vi "test_Error Code and Message Status Channels by Generating TCP Errors.vi"(8 "error in (no error)":errorcluster, 11 "TestCase in":refnum<class "Instrument Addon Error System Tests.lvclass">) -> (0 "error out":errorcluster, 3 "TestCase out":refnum<class "Instrument Addon Error System Tests.lvclass">)   [LabVIEW 2019, in "Instrument Addon Error System Tests.lvclass"]
uses:
  Instrument Addon Error System Tests.lvclass
  C:/Program Files (x86)/National Instruments/LabVIEW 2019/vi.lib/NI/VeriStand Custom Device Testing Tools/VeriStandTestCase/VeriStandTestCase.lvclass
  <vilib>/NI VeriStand/Execution/Workspace/NI VeriStand - Set Multiple Channel Values.vi
  <vilib>/NI VeriStand/Execution/Workspace/NI VeriStand - Get Single Channel Value.vi
  <vilib>/addons/_JKI Toolkits/VI Tester/TestCase.llb/TestCase.lvclass
  <vilib>/NI VeriStand/Execution/Workspace/NI_VS Workspace ExecutionAPI.lvlib
  C:/Program Files (x86)/National Instruments/LabVIEW 2019/vi.lib/addons/_JKI Toolkits/VI Tester/TestCase.llb/TestCase.lvclass
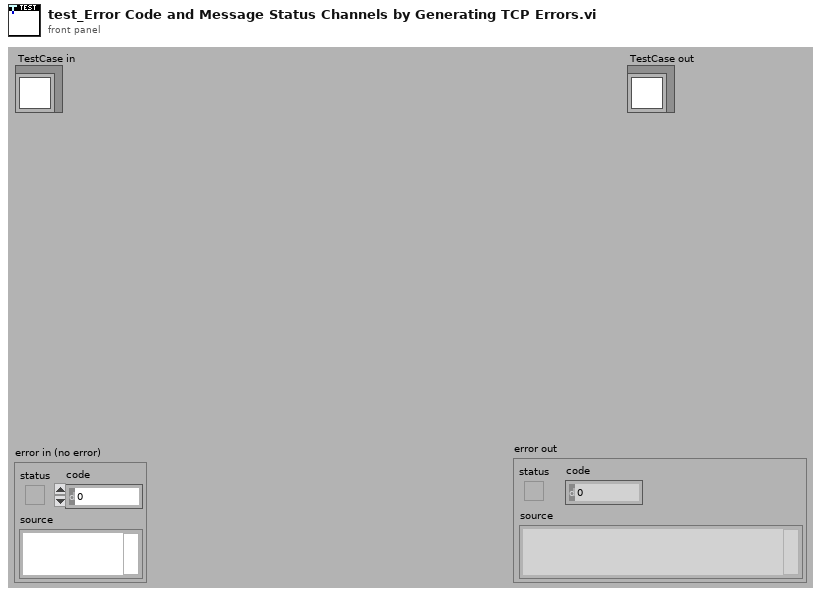
[diagram p1: front panel]
types:
  T1 = typedef "NI_VS Workspace ExecutionAPI.lvlib/WorkspaceAPI.ctl" = refnum<k24>
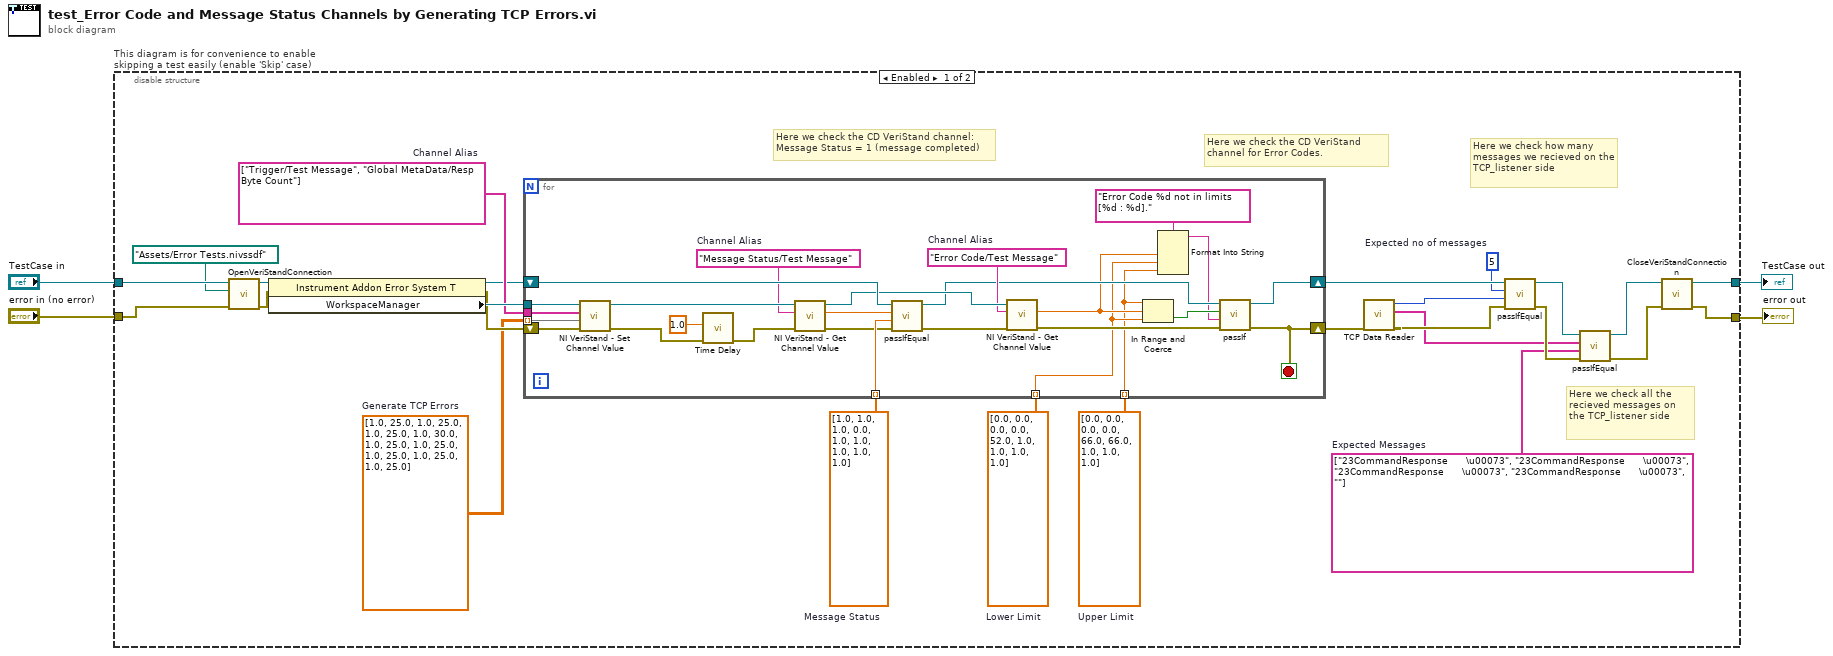
[diagram p0: block diagram]
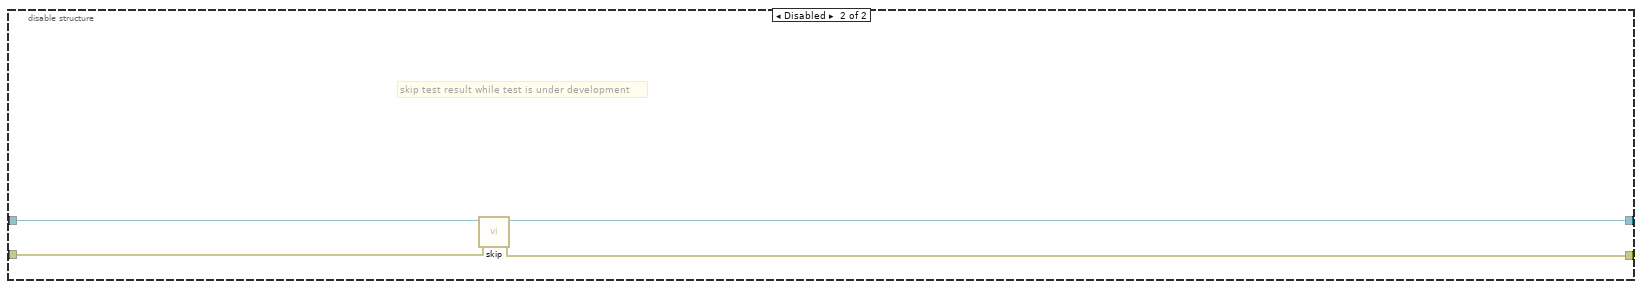
[diagram p2: hidden frame]
diagram:
  n1 = disable-structure "This diagram is for convenience to enable skipping a test easily (enable 'Skip' case)" shown="Enabled" {
    disable-tunnel: "TestCase in" -> [w28 w60]
    disable-tunnel: [w29 w58] -> w1
    disable-tunnel: [w30 w59] -> w3
    disable-tunnel: "error in (no error)" -> [w26 w57]
    frame Enabled {
      w5 = dbl[] [0.0, 0.0, 0.0, 0.0, 52.0, 1.0, 1.0, 1.0, 1.0]  # Lower Limit
      w6 = dbl[] [0.0, 0.0, 0.0, 0.0, 66.0, 66.0, 1.0, 1.0, 1.0]  # Upper Limit
      w7 = dbl[] [1.0, 1.0, 1.0, 0.0, 1.0, 1.0, 1.0, 1.0, 1.0]  # Message Status
      w8 = dbl[][] [[1.0, 25.0], [1.0, 25.0], [1.0, 25.0], [1.0, 30.0], [1.0, 25.0], [1.0, 25.0], [1.0, 25.0], [1.0, 25.0], [1.0, 25.0]]  # Generate TCP Errors
      w14 = string[] ["23CommandResponse      \u00073", "23CommandResponse      \u00073", "23CommandResponse      \u00073", "23CommandResponse      \u00073", ""]  # Expected Messages
      w13 = 5  # Expected no of messages
      w21 = string[] ["Trigger/Test Message", "Global MetaData/Resp Byte Count"]  # Channel Alias
      # "Here we check the CD VeriStand channel:\nMessage Status = 1 (message completed)"
      # "Here we check the CD VeriStand channel for Error Codes."
      # "Here we check all the recieved messages on the TCP_listener side"
      # "Here we check how many messages we recieved on the TCP_listener side"
      n2 = call-dynamic "OpenVeriStandConnection.vi"("error in (no error)"=w26, "System Definition File"=path "Assets/Error Tests.nivssdf", "VeriStand Test Case in"=w28) -> ("error out"=w25:errorcluster, "VeriStand Test Case out"=w27:refnum<class "Instrument Addon Error System Tests.lvclass">)  [unwired: 6 in, 1 out]
      n3 = property class="Instrument Addon Error System T"(reference=w27, error in=w25) -> (reference out=w20:refnum<class "Instrument Addon Error System Tests.lvclass">, error out=w22:errorcluster, "WorkspaceManager"=w23:T1)
      n4 = for {
        tunnel: w23 -> [w56]
        tunnel: w21 -> [w54]
        tunnel: w8 -> [w52] mode=indexing
        shift-right: [w37] -> w12
        shift-left: w22 -> [w55]
        shift-right: [w40] -> w15
        shift-left: w20 -> [w53]
        tunnel: w7 -> [w47] mode=indexing
        tunnel: w6 -> [w31] mode=indexing
        tunnel: w5 -> [w32] mode=indexing
        stop <- w37 stop-if-true
        w42 = "Error Code/Test Message"  # Channel Alias
        w45 = "Message Status/Test Message"  # Channel Alias
        n5 = call-poly <vilib>:"NI VeriStand - Set Channel Value.vi"("error in (no error)"=w55, "Values"=w52, "Channels"=w54, "WorkspaceManager in"=w56) -> ("error out"=w48:errorcluster, "WorkspaceManager out"=w49:T1)  [unwired: 6 in]
        n6 = call "Time Delay"("error in (no error)"=w48, "Delay Time (s)"=1.0) -> ("error out"=w50:errorcluster)  [unwired: 9 in]
        n7 = call-poly <vilib>:"NI VeriStand - Get Channel Value.vi"("error in (no error)"=w50, "Channel"=w45, "WorkspaceManager in"=w49) -> ("error out"=w44:errorcluster, "Value"=w46:dbl, "WorkspaceManager out"=w43:T1)  [unwired: 6 in]
        n8 = call-dynamic "passIfEqual.vi"("error in (no error)"=w44, "y"=w47, "x"=w46, "TestCase in"=w53) -> ("error out"=w38:errorcluster, "TestCase out"=w41:refnum<class "Instrument Addon Error System Tests.lvclass">)  [unwired: 6 in]
        n9 = call-poly <vilib>:"NI VeriStand - Get Channel Value.vi"("error in (no error)"=w38, "Channel"=w42, "WorkspaceManager in"=w43) -> ("error out"=w39:errorcluster, "Value"=w33:dbl)  [unwired: 6 in, 1 out]
        n10 = In Range and Coerce(upper limit=w31, x=w33, lower limit=w32) -> (In Range?=w36:bool)  [unwired: 1 out]
        n11 = Format Into String(format string="Error Code %d not in limits [%d : %d]." ("message (\"\")"), w33, w32, w31) -> (resulting string=w35:string)  [unwired: 2 in, 1 out]
        n12 = call-dynamic "passIf.vi"("error in (no error)"=w39, "message (\"\")"=w35, "pass"=w36, "TestCase in"=w41) -> ("error out"=w37:errorcluster, "TestCase out"=w40:refnum<class "Instrument Addon Error System Tests.lvclass">)  [unwired: 6 in]
      }
      n13 = call "TCP Data Reader.vi"("error in (no error)"=w12) -> ("error out"=w10:errorcluster, "Recieved Messages"=w9:string[], "No of messages"=w11:i32)  [unwired: 8 in]
      n14 = call-dynamic "passIfEqual.vi"("error in (no error)"=w10, "y"=w11, "x"=w13, "TestCase in"=w15) -> ("error out"=w17:errorcluster, "TestCase out"=w19:refnum<class "Instrument Addon Error System Tests.lvclass">)  [unwired: 6 in]
      n15 = call-dynamic "passIfEqual.vi"("error in (no error)"=w17, "y"=w14, "x"=w9, "TestCase in"=w19) -> ("error out"=w16:errorcluster, "TestCase out"=w18:refnum<class "Instrument Addon Error System Tests.lvclass">)  [unwired: 6 in]
      n16 = call-dynamic "CloseVeriStandConnection.vi"("error in (no error)"=w16, "VeriStand Test Case in"=w18) -> ("error out"=w30:errorcluster, "VeriStand Test Case out"=w29:refnum<class "Instrument Addon Error System Tests.lvclass">)  [unwired: 8 in]
    }
    frame Disabled {
      # "skip test result while test is under development"
      n17 = call <vilib>:"skip.vi"("error in (no error)"=w57, "TestCase in"=w60) -> ("error out"=w59:errorcluster, "TestCase out"=w58:refnum<class "Instrument Addon Error System Tests.lvclass">)  [unwired: 8 in]
    }
  }
  "error out" <- w3
  "TestCase out" <- w1
